vi "Set_DB.vi"(8 "error in (no error)":errorcluster, 11 "Control-Server in":refnum<class "Control-Server.lvclass">) -> (0 "error out":errorcluster, 3 "Control-Server out":refnum<class "Control-Server.lvclass">)   [LabVIEW 2015, in "Control-Server.lvclass"]
uses:
  Control-Server.lvclass
  Config/config_names_def.ctl
  dependecies/ControlsVIs/Clusters-def/Message types.ctl
  Message/Message.lvclass
  Control-Server.lvclass/Control-Server.ctl
  DB/DB_MySQL/DB_MySQL.lvclass
  DB/DB_SQLite/DB_SQLite.lvclass
  Message/Message.lvclass/Message.ctl
  GeneralFunctionality/GeneralFunctionality.lvclass/GeneralFunctionality.ctl
  DB/DB.lvclass/DB.ctl
  Config/Config.lvclass
  GeneralFunctionality/GeneralFunctionality.lvclass
  DB/DB.lvclass
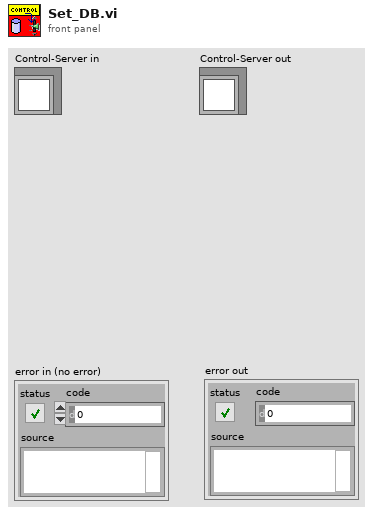
[diagram p1: front panel]
types:
  T1 = typedef "Config.lvclass/config_names_def.ctl" = string
  T2 = typedef "Message types.ctl" = string
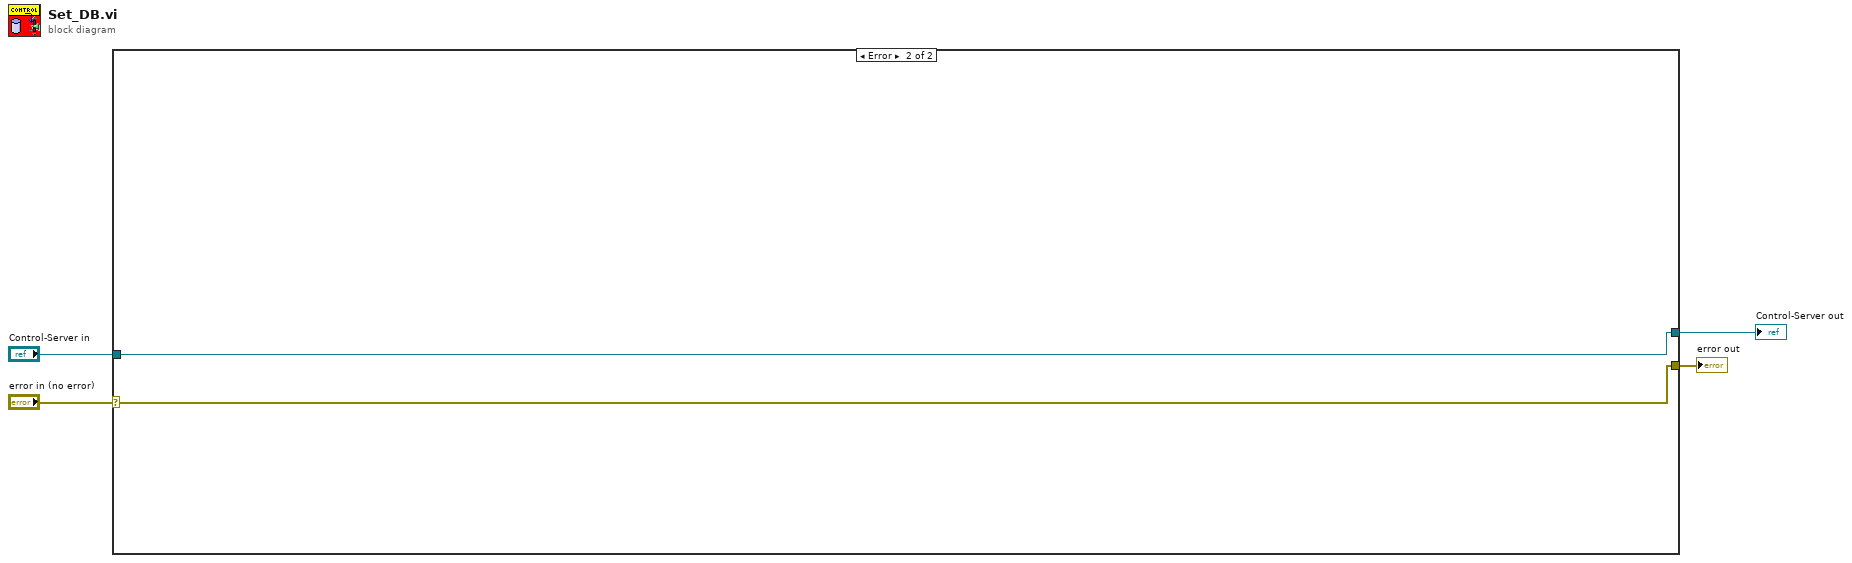
[diagram p0: block diagram]
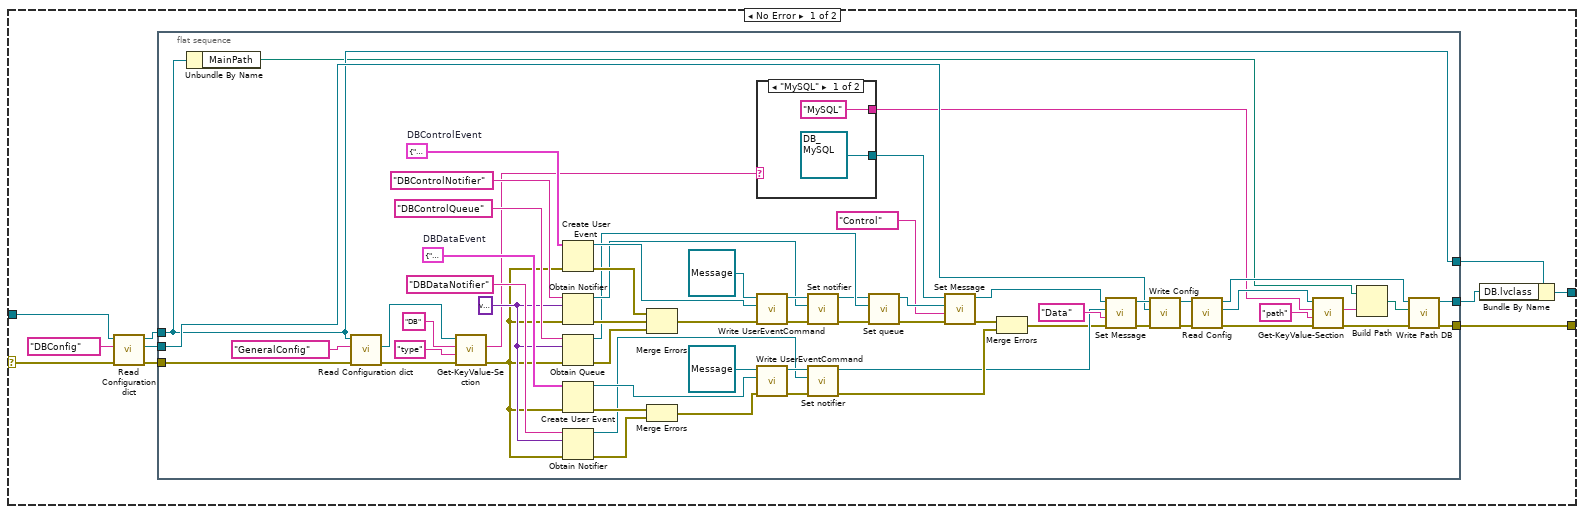
[diagram p2: hidden frame]
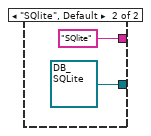
[diagram p3: hidden frame]
diagram:
  n1 = case shown="Error" "error in (no error)" {
    selector: "error in (no error)" -> [w6 w81]
    tunnel: [w12 w81] -> w4
    tunnel: "Control-Server in" -> [w11 w80]
    tunnel: [w5 w80] -> w1
    frame No Error {
      n2 = call "Read Configuration dict.vi"("error in (no error)"=w6, "Config Name"=T1 "DBConfig", "Control in"=w11) -> ("error out"=w10:errorcluster, "Config"=w14:refnum<class "Config.lvclass">, "Control out"=w9:refnum<class "Control-Server.lvclass">)  [unwired: 6 in]
      n3 = flat-sequence {
        tunnel: w10 -> [w32]
        tunnel: [w22] -> w12
        tunnel: w14 -> [w45]
        tunnel: w9 -> [w18]
        tunnel: [w21] -> w8
        tunnel: [w18] -> w7
        frame #0 {
          w38 = variant
          w65 = cluster{"command":string, "data":variant} {"command"="", "data"=variant}  # DBDataEvent
          w71 = cluster{"command":string, "data":variant} {"command"="", "data"=variant}  # DBControlEvent
          n4 = Unbundle By Name(w18) -> ("MainPath"=w17:path)
          n5 = call "Read Configuration dict.vi"("error in (no error)"=w32, "Config Name"=T1 "GeneralConfig", "Control in"=w18) -> ("error out"=w31:errorcluster, "Config"=w35:refnum<class "Config.lvclass">)  [unwired: 6 in, 1 out]
          n6 = call-dynamic "Get-KeyValue-Section.vi"("error in (no error)"=w31, "Key"="type", "Section"="DB", "Config in"=w35) -> ("error out"=w30:errorcluster, "Value"=w29:string)  [unwired: 5 in, 1 out]
          n7 = Create User Event(user event datatype=w71, error in=w30) -> (user event=w73:refnum<user-event>, error out=w69:errorcluster)
          n8 = Obtain Notifier(name (unnamed)="DBControlNotifier" ("nom (aucun)"), notification data type=w38, error in (no error)=w30) -> (notifier out=w67:refnum<notifier>, error out=w68:errorcluster)  [unwired: 1 in, 1 out]
          n9 = Obtain Queue(name (unnamed)="DBControlQueue", element data type=w38, error in (no error)=w30) -> (queue out=w53:refnum<queue>, error out=w52:errorcluster)  [unwired: 2 in, 1 out]
          n10 = Create User Event(user event datatype=w65, error in=w30) -> (user event=w62:refnum<user-event>, error out=w59:errorcluster)
          n11 = Obtain Notifier(name (unnamed)="DBDataNotifier" ("nom (aucun)"), notification data type=w38, error in (no error)=w30) -> (notifier out=w57:refnum<notifier>, error out=w58:errorcluster)  [unwired: 1 in, 1 out]
          n12 = Merge Errors(w69, w68, w52) -> (w66:errorcluster)
          n13 = Merge Errors(w59, w58) -> (w56:errorcluster)
          n14 = case shown="\"MySQL\"" w29 {
            tunnel: [refnum<class "DB_MySQL.lvclass"> refnum ("DB_MySQL.lvclass") refnum<class "DB_SQLite.lvclass"> refnum ("DB_SQLite.lvclass")] -> w37
            tunnel: ["MySQL" "SQlite"] -> w15
            frame "MySQL" {
            }
            frame "SQlite", Default {
            }
          }
          n15 = call "Write UserEventCommand.vi"("error in (no error)"=w66, "UserEventCommand"=w73, "Message en entrée"=refnum<class "Message.lvclass"> refnum ("Message.lvclass")) -> ("error out"=w70:errorcluster, "Message en sortie"=w74:refnum<class "Message.lvclass">)  [unwired: 7 in]
          n16 = call "Write UserEventCommand.vi"("error in (no error)"=w56, "UserEventCommand"=w62, "Message en entrée"=refnum<class "Message.lvclass"> refnum ("Message.lvclass")) -> ("error out"=w60:errorcluster, "Message en sortie"=w61:refnum<class "Message.lvclass">)  [unwired: 7 in]
          n17 = call "Set notifier.vi"("error in (no error)"=w70, "notifier"=w67, "Message en entrée"=w74) -> ("error out"=w51:errorcluster, "Message en sortie"=w50:refnum<class "Message.lvclass">)  [unwired: 7 in]
          n18 = call "Set notifier.vi"("error in (no error)"=w60, "notifier"=w57, "Message en entrée"=w61) -> ("error out"=w55:errorcluster, "Message en sortie"=w43:refnum<class "Message.lvclass">)  [unwired: 7 in]
          n19 = call "Set queue.vi"("error in (no error)"=w51, "queue"=w53, "Message in"=w50) -> ("error out"=w39:errorcluster, "Message out"=w49:refnum<class "Message.lvclass">)  [unwired: 7 in]
          n20 = call "Set Message.vi"("error in (no error)"=w39, "Message type"=T2 "Control", "Message.lvclass"=w49, "GeneralFunctionality en entrée"=w37) -> ("error out"=w42:errorcluster, "GeneralFunctionality en sortie"=w47:refnum<class "DB.lvclass">)  [unwired: 6 in]
          n21 = Merge Errors(w42, w55) -> (w41:errorcluster)
          n22 = call "Set Message.vi"("error in (no error)"=w41, "Message type"=T2 "Data", "Message.lvclass"=w43, "GeneralFunctionality en entrée"=w47) -> ("error out"=w40:errorcluster, "GeneralFunctionality en sortie"=w46:refnum<class "DB.lvclass">)  [unwired: 6 in]
          n23 = call "Write Config.vi"("error in (no error)"=w40, "Config.lvclass"=w45, "GeneralFunctionality en entrée"=w46) -> ("error out"=w19:errorcluster, "GeneralFunctionality en sortie"=w25:refnum<class "DB.lvclass">)  [unwired: 7 in]
          n24 = call "Read Config.vi"("error in (no error)"=w19, "GeneralFunctionality en entrée"=w25) -> ("error out"=w28:errorcluster, "Config.lvclass"=w27:refnum<class "Config.lvclass">, "GeneralFunctionality en sortie"=w20:refnum<class "DB.lvclass">)  [unwired: 7 in]
          n25 = call-dynamic "Get-KeyValue-Section.vi"("error in (no error)"=w28, "Key"="path", "Section"=w15, "Config in"=w27) -> ("error out"=w23:errorcluster, "Value"=w26:string)  [unwired: 5 in, 1 out]
          n26 = Build Path(base path=w17, name or relative path=w26) -> (appended path=w24:path)
          n27 = call "Write Path DB.vi"("error in (no error)"=w23, "Path DB"=w24, "DB in"=w20) -> ("error out"=w22:errorcluster, "DB out"=w21:refnum<class "DB.lvclass">)  [unwired: 7 in]
        }
      }
      n28 = Bundle By Name(cluster=w7, "DB.lvclass"=w8) -> (w5:refnum<class "Control-Server.lvclass">)
    }
    frame Error {
    }
  }
  "error out" <- w4
  "Control-Server out" <- w1
